vi "Get Next Bus Engine State.vi"(8 "error in (no error)":errorcluster, 10 "Bus State":T3, 11 "Cmd Q":refnum<queue>) -> (0 "error out":errorcluster, 2 "Bus State":T3, 3 "Command Cluster":T1)   [LabVIEW 2019, in "CAN Stream Support Workspace Shared.lvlib"]
uses:
  CAN Stream Support Workspace Shared.lvlib
  Types/Host Stream Engine State.ctl
  Types/Host Stream Queue Type.ctl
  Types/Host Stream Queue Command.ctl
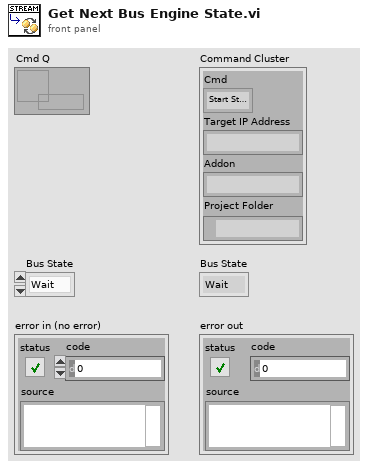
[diagram p1: front panel]
types:
  T1 = typedef "CAN Stream Support Workspace Shared.lvlib/Host Stream Queue Type.ctl" = cluster{"Cmd":T2, "Target IP Address":string, "Addon":string, "Project Folder":path}
  T2 = typedef "CAN Stream Support Workspace Shared.lvlib/Host Stream Queue Command.ctl" = enum8{"Start Stream", "Stop Stream", "Exit"}
  T3 = typedef "CAN Stream Support Workspace Shared.lvlib/Host Stream Engine State.ctl" = enum8{"Wait", "Start Stream", "Read Stream", "Stop Stream", "Exit"}
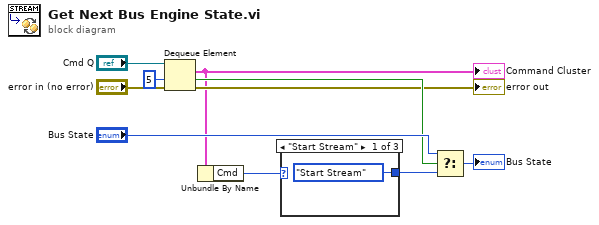
[diagram p0: block diagram]
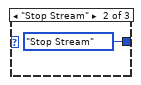
[diagram p2: hidden frame]
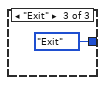
[diagram p3: hidden frame]
diagram:
  n1 = Dequeue Element(queue="Cmd Q", timeout in ms (-1)=5, error in (no error)="error in (no error)") -> (element=w3:T1, timed out?=w7:bool, error out=→"error out":errorcluster)  [unwired: 1 out]
  "Command Cluster" <- w3
  n2 = Unbundle By Name(w3) -> ("Cmd"=w2:T2)
  n3 = case shown="\"Start Stream\"" w2 {
    tunnel: [Host_Stream_Engine_State."Start Stream" Host_Stream_Engine_State."Stop Stream" Host_Stream_Engine_State."Exit"] -> w1
    frame "Start Stream" {
    }
    frame "Stop Stream" {
    }
    frame "Exit" {
    }
  }
  n4 = Select(t="Bus State", s=w7, f=w1) -> (s? t:f=→"Bus State":T3)
